vi "II region controlls.vi"() -> ()   [LabVIEW 2017]
uses:
  <instrlib>/BK Precision 913XX/BK Precision 913XX.lvlib
panel:
  out "Actual Voltage Level (V) 3":dbl format="%.4g"
  out "Actual Power Level (W) 3":dbl format="%.4g"
  out "Actual Current Level (A) 3":dbl format="%.4g"
  out "Actual Voltage Level (V) 2":dbl format="%.4g"
  out "Actual Power Level (W) 2":dbl format="%.4g"
  out "Actual Current Level (A) 2":dbl format="%.4g"
  in  "Voltage Level (0.0 V) 3":dbl format="%.3g"
  in  "Voltage Level (0.0 V) 2":dbl format="%.3g"
  in  "Channel (3:3)":u16(ring)=1 items=["1"=1, "2"=2, "3"=3]
  in  "Channel (2:2)":u16(ring)=1 items=["1"=1, "2"=2, "3"=3]
  in  "Voltage Level (0.0 V)":dbl format="%.3g"
  in  "Voltage Limit (36.000 V)":dbl=36.0 min=0.0 max=66.0 step=0.001 format="%.3g"
  in  "Enable OVP (T: Enable)":bool=TRUE
  in  "Channel (1:1)":u16(ring)=1 items=["1"=1, "2"=2, "3"=3]
  in  "Current Limit (0.0 A)":dbl min=0.0 max=25.0 step=1.0 format="%.3f"
  in  "Stop Output":bool
  out "Actual Current Level (A)":dbl format="%.4g"
  out "Actual Power Level (W)":dbl format="%.4g"
  out "Actual Voltage Level (V)":dbl format="%.4g"
  in  "VISA resource name":refnum<visa-resource-name>
  # "C H A N N E L  0 3"
  # "C H A N N E L  0 1"
  # "C H A N N E L  0 2"
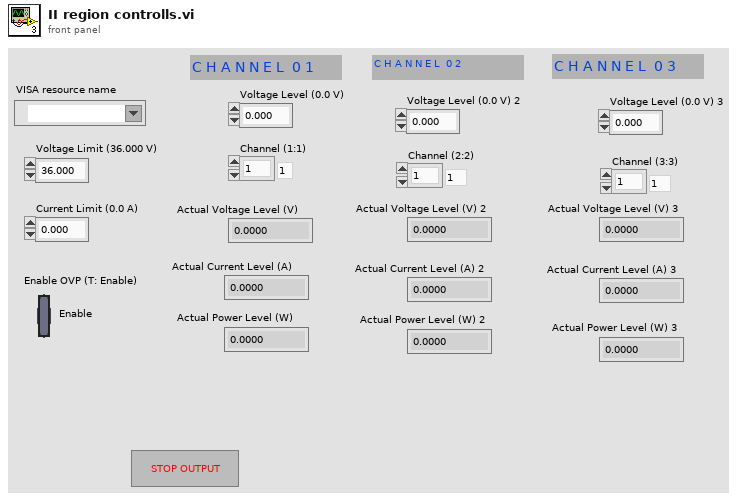
[diagram p1: front panel]
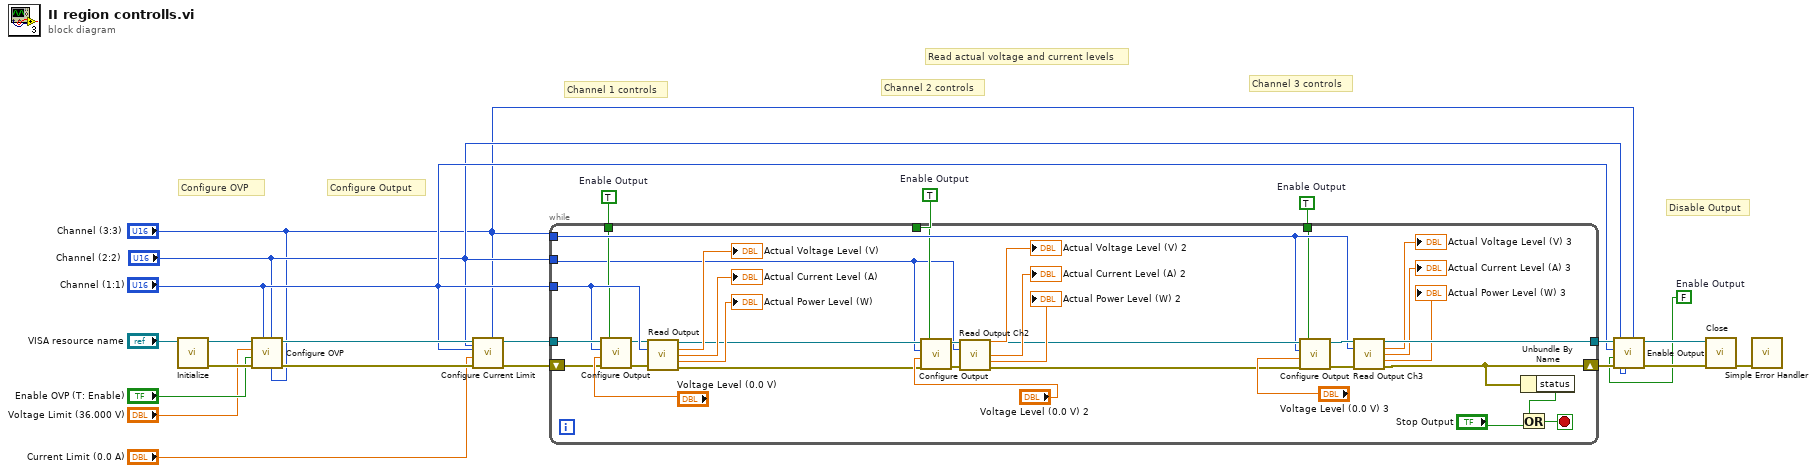
[diagram p0: block diagram]
diagram:
  w3 = TRUE  # Enable Output
  w4 = TRUE  # Enable Output
  w5 = TRUE  # Enable Output
  w7 = FALSE  # Enable Output
  # "Channel 3 controls"
  # "Channel 2 controls"
  # "Channel 1 controls"
  # "Disable Output"
  # "Read actual voltage and current levels"
  # "Configure Output"
  # "Configure OVP"
  n1 = call <instrlib>:"Initialize.vi"("VISA resource name"="VISA resource name") -> ("error out"=w20:errorcluster, "VISA resource name out"=w19:refnum<visa-resource-name>)  [unwired: 9 in]
  n2 = call <instrlib>:"Configure OVP.vi"("Channel (3:3)"="Channel (3:3)", "Channel (2:2)"="Channel (2:2)", "Channel (1:1)"="Channel (1:1)", "error in (no error)"=w20, "Enable OVP (T: Enable)"="Enable OVP (T: Enable)", "Voltage Limit (36.000 V)"="Voltage Limit (36.000 V)", "VISA resource name"=w19) -> ("error out"=w17:errorcluster, "VISA resource name out"=w18:refnum<visa-resource-name>)  [unwired: 3 in]
  n3 = call <instrlib>:"Configure Current Limit.vi"("Channel (3:3)"="Channel (3:3)", "Channel (2:2)"="Channel (2:2)", "error in (no error)"=w17, "Current Limit (0.0 A)"="Current Limit (0.0 A)", "Channel (1:1)"="Channel (1:1)", "VISA resource name"=w18) -> ("error out"=w13:errorcluster, "VISA resource name out"=w12:refnum<visa-resource-name>)  [unwired: 4 in]
  n4 = while {
    tunnel: w12 -> [w51]
    tunnel: [w48] -> w16
    shift-right: [w24] -> w11
    shift-left: w13 -> [w30]
    tunnel: "Channel (1:1)" -> [w50]
    tunnel: "Channel (2:2)" -> [w23]
    tunnel: "Channel (3:3)" -> [w37]
    tunnel: w5 -> [w36]
    tunnel: w4 -> [w32]
    tunnel: w3 -> [w35]
    stop <- w57 stop-if-true
    n5 = call <instrlib>:"Configure Output.vi"("Enable Channel Output (F: False)"=w36, "error in (no error)"=w30, "Voltage Level (0.0 V)"="Voltage Level (0.0 V)", "Channel (1:1)"=w50, "VISA resource name"=w51) -> ("error out"=w29:errorcluster, "VISA resource name out"=w40:refnum<visa-resource-name>)  [unwired: 5 in]
    n6 = call <instrlib>:"Read Output.vi"("VISA resource name"=w40, "Channel (1:Channel 1)"=w50, "error in (no error)"=w29) -> ("VISA resource name out"=w33:refnum<visa-resource-name>, "Actual Voltage Level (V)"=→"Actual Voltage Level (V)":dbl, "Actual Current Level (A)"=→"Actual Current Level (A)":dbl, "Actual Power Level (W)"=→"Actual Power Level (W)":dbl, "error out"=w28:errorcluster)  [unwired: 8 in]
    n7 = call <instrlib>:"Configure Output.vi"("Enable Channel Output (F: False)"=w32, "error in (no error)"=w28, "Voltage Level (0.0 V)"="Voltage Level (0.0 V) 2", "Channel (1:1)"=w23, "VISA resource name"=w33) -> ("error out"=w27:errorcluster, "VISA resource name out"=w34:refnum<visa-resource-name>)  [unwired: 5 in]
    n8 = call <instrlib>:"Read Output Ch2.vi"("VISA resource name"=w34, "Channel (1:Channel 1)"=w23, "error in (no error)"=w27) -> ("VISA resource name out"=w39:refnum<visa-resource-name>, "Actual Voltage Level (V)"=→"Actual Voltage Level (V) 2":dbl, "Actual Current Level (A)"=→"Actual Current Level (A) 2":dbl, "Actual Power Level (W)"=→"Actual Power Level (W) 2":dbl, "error out"=w26:errorcluster)  [unwired: 8 in]
    n9 = call <instrlib>:"Configure Output.vi"("Enable Channel Output (F: False)"=w35, "error in (no error)"=w26, "Voltage Level (0.0 V)"="Voltage Level (0.0 V) 3", "Channel (1:1)"=w37, "VISA resource name"=w39) -> ("error out"=w25:errorcluster, "VISA resource name out"=w38:refnum<visa-resource-name>)  [unwired: 5 in]
    n10 = call <instrlib>:"Read Output Ch3.vi"("VISA resource name"=w38, "Channel (1:Channel 1)"=w37, "error in (no error)"=w25) -> ("VISA resource name out"=w48:refnum<visa-resource-name>, "Actual Voltage Level (V)"=→"Actual Voltage Level (V) 3":dbl, "Actual Current Level (A)"=→"Actual Current Level (A) 3":dbl, "Actual Power Level (W)"=→"Actual Power Level (W) 3":dbl, "error out"=w24:errorcluster)  [unwired: 8 in]
    n11 = Unbundle By Name(w24) -> ("status"=w55:bool)
    n12 = Or(x=w55, y="Stop Output") -> (x .or. y?=w57:bool)
  }
  n13 = call <instrlib>:"Enable Output.vi"("Channel (3:3)"="Channel (3:3)", "Channel (2:2)"="Channel (2:2)", "error in (no error)"=w11, "Enable Output (F: False)"=w7, "Channel (1:1)"="Channel (1:1)", "VISA resource name"=w16) -> ("error out"=w14:errorcluster, "VISA resource name out"=w15:refnum<visa-resource-name>)  [unwired: 4 in]
  n14 = call <instrlib>:"Close.vi"("error in (no error)"=w14, "VISA resource name"=w15) -> ("error out"=w21:errorcluster)  [unwired: 9 in]
  n15 = call <vilib>:"Simple Error Handler.vi"("error in (no error)"=w21) -> ()  [unwired: 4 in, 5 out]
